vi "Toggle (SubVI).vi"(6 "Button 1":bool, 7 "Shifter On in":bool, 9 "HasPressedShifterButton":bool, 10 "reference in":refnum<vi>, 11 "Boolean in":refnum<vi>) -> (3 "Shifter On out":bool)   [LabVIEW 2012]
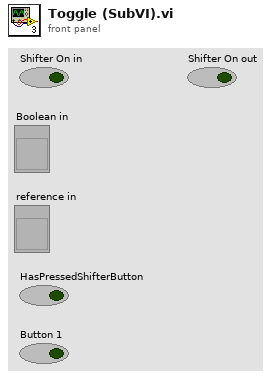
[diagram p1: front panel]
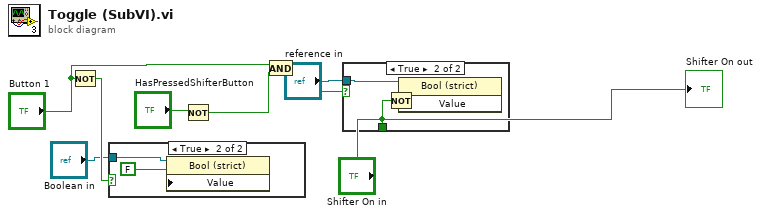
[diagram p0: block diagram]
diagram:
  n1 = Not(x="Button 1") -> (.not. x?=w5:bool)
  n2 = case shown="True" w5 {
    tunnel: "Boolean in" -> [_ w9]
    frame False {
    }
    frame True {
      n3 = property class="Bool (strict)"(reference=w9, "Value"=FALSE ("HasPressedArmsButton")) -> ()  [unwired: 1 in, 2 out]
    }
  }
  n4 = Not(x="HasPressedShifterButton") -> (.not. x?=w4:bool)
  n5 = And(x="Button 1", y=w4) -> (x .and. y?=w6:bool)
  n6 = case shown="True" w6 {
    tunnel: "Shifter On in" -> [_ w12]
    tunnel: "reference in" -> [_ w11]
    frame False {
    }
    frame True {
      n7 = Not(x=w12) -> (.not. x?=w13:bool)
      n8 = property class="Bool (strict)"(reference=w11, "Value"=w13) -> ()  [unwired: 1 in, 2 out]
    }
  }
  "Shifter On out" <- "Shifter On in"
